vi "BuildPlaylist.vi"(3 "playlist":string="Current.txt") -> ()   [LabVIEW 2010]
uses:
  SlideParams.ctl
  <vilib>/Utility/file.llb/Read From Spreadsheet File (string).vi
  <vilib>/Utility/file.llb/Write To Spreadsheet File (string).vi
  <vilib>/Utility/cursorutil.llb/Set Cursor (Icon Pict).vi
panel:
  out "last last lineup":string[][](array[string])
  out "last lineup":string[][](array[string])
  out "Moving":bool
  in  "Revert":bool
  in  "Preview":bool
  in  "Save As":bool
  in  "Undo":bool
  out "location":cluster{dbl, dbl}
  out "Offset":cluster{"X":i32, "Y":i32}
  out "slide":i32
  in  "Tab Control":enum32{"Table", "Map", "LUT"}(tab)=enum."Map"
  in  "Table Control":string[][](table)
  out "Total":i32
  in  "ZOOM":dbl(slide) scale=0.1..2.0
  out "Slide":picture
  out "2D Map":picture
  in  "iterator":i32
  in  "Mod":T1=enum."Bounce"
  out "LUT":T2(array[cluster])
  in  "Save":bool
  # "/"
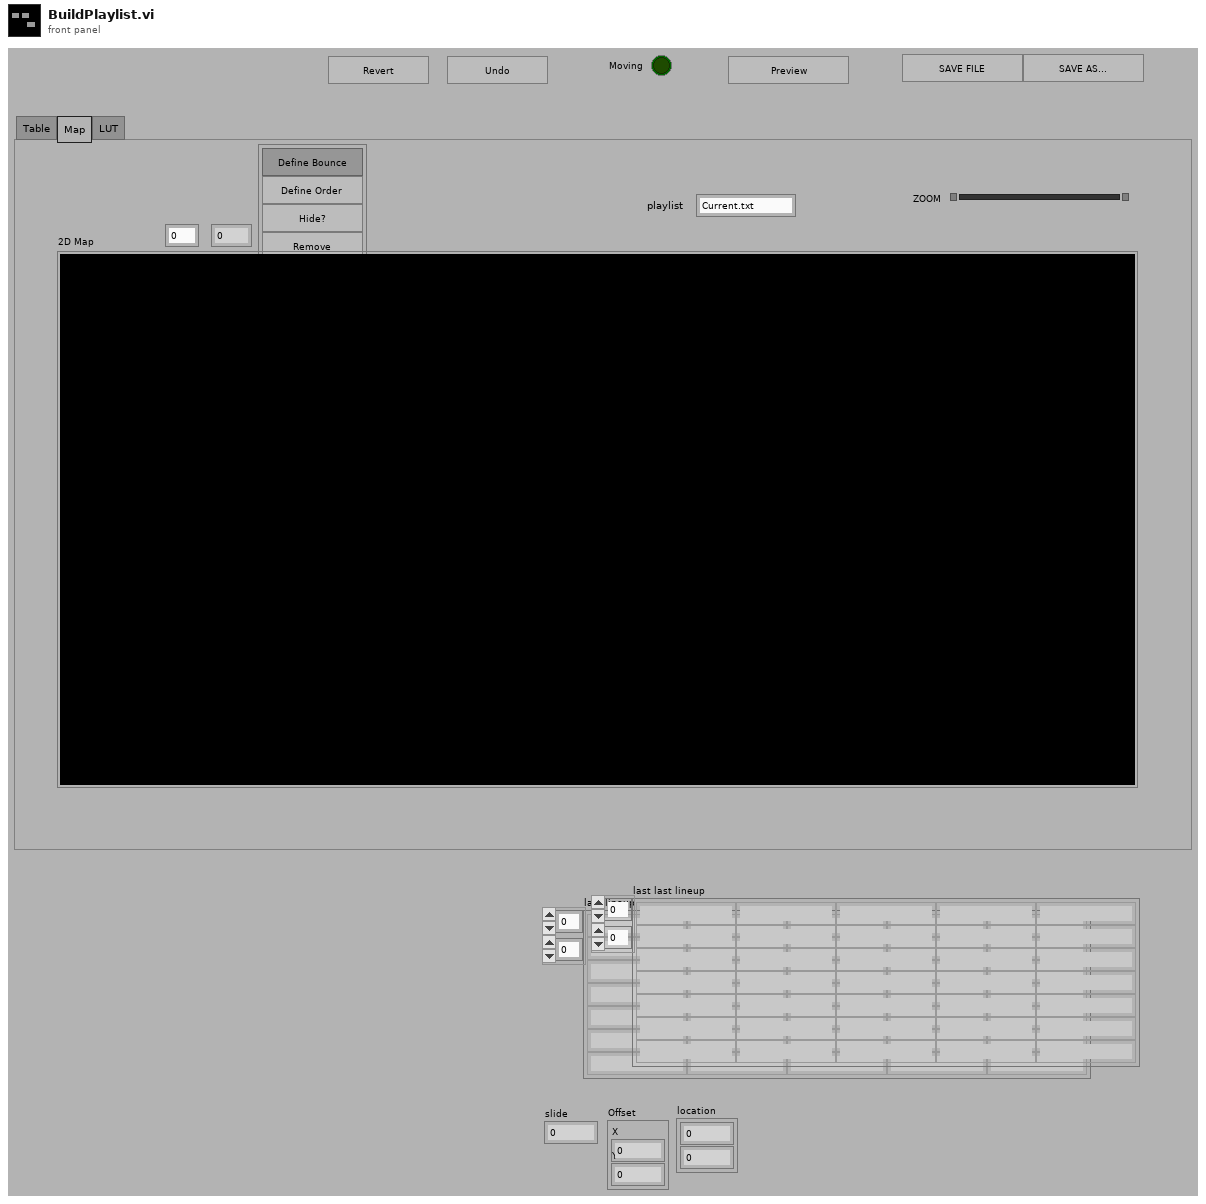
[diagram p1: front panel]
types:
  T1 = typedef "SlideParams.ctl" = enum32{"No Selection", "Bounce", "Order", "Hide", "Remove"}
  T2 = cluster{"col":i32, "row":i32, "rect":cluster{"left":i16, "top":i16, "right":i16, "bottom":i16}, "Name":string}[]
  T3 = typedef "LVPoint32TypeDef.ctl" = cluster{"Horizontal":i32, "Vertical":i32}
  T4 = typedef "LVMouseTypeDef.ctl" = cluster{"Mouse Position":cluster{"X":i32, "Y":i32}, "Mouse Modifiers":cluster{"Button Down":bool, "Shift Mod":bool, "Menu Mod":bool, "Option Mod":bool}}
  T5 = typedef "LVPointTypeDef.ctl" = cluster{"Horizontal":i16, "Vertical":i16}
  T6 = typedef "LVPositionTypeDef.ctl" = cluster{"Left":i32, "Top":i32}
  T7 = cluster{"col":i32, "row":i32, "rect":cluster{"left":i16, "top":i16, "right":i16, "bottom":i16}, "Name":string}
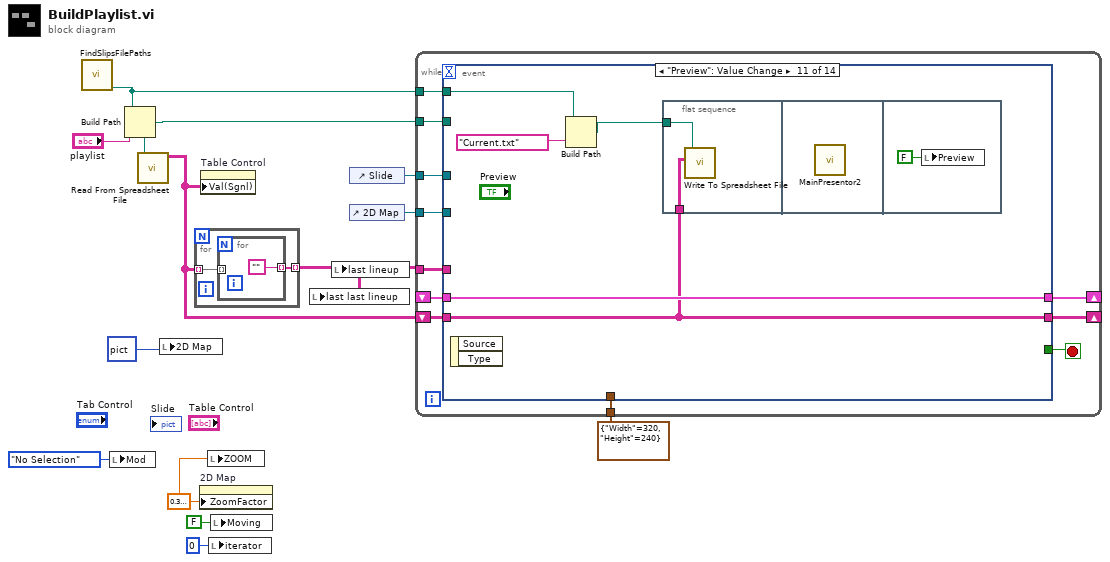
[diagram p0: block diagram]
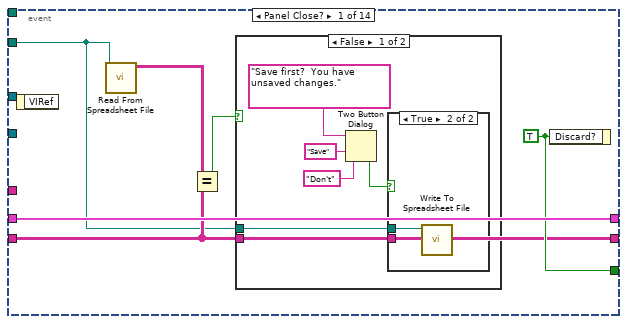
[diagram p2: hidden frame]
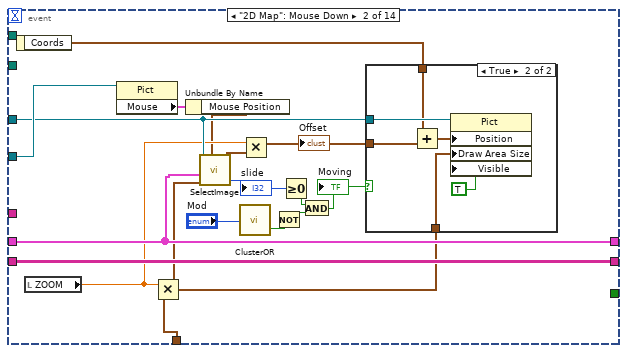
[diagram p5: hidden frame]
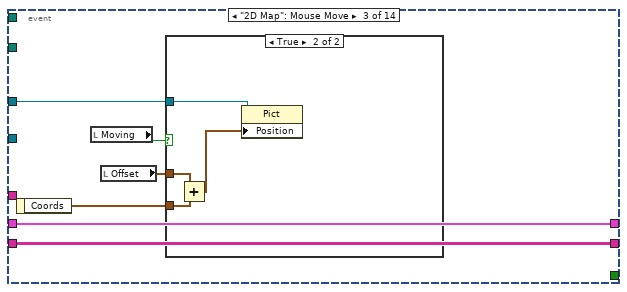
[diagram p7: hidden frame]
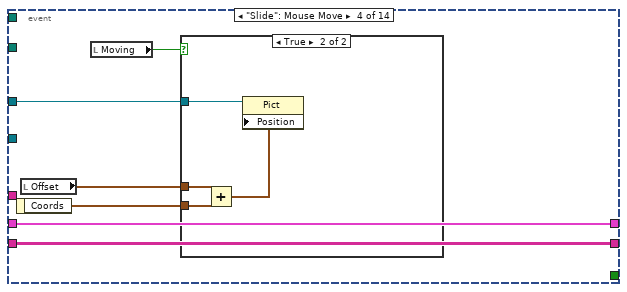
[diagram p9: hidden frame]
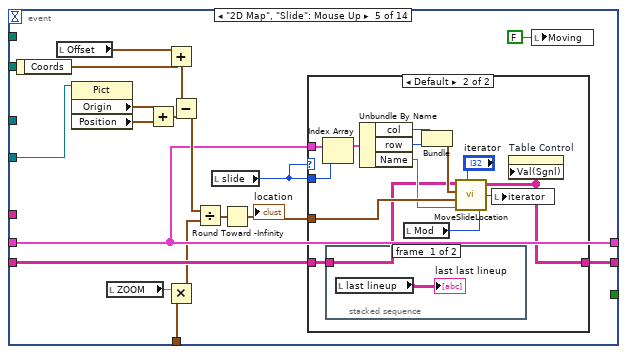
[diagram p11: hidden frame]
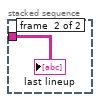
[diagram p13: hidden frame]
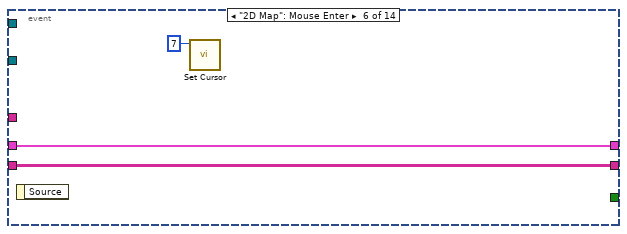
[diagram p14: hidden frame]
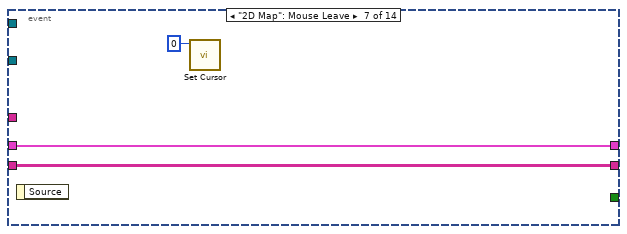
[diagram p15: hidden frame]
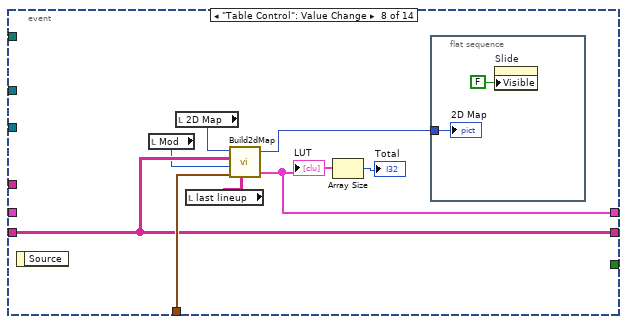
[diagram p16: hidden frame]
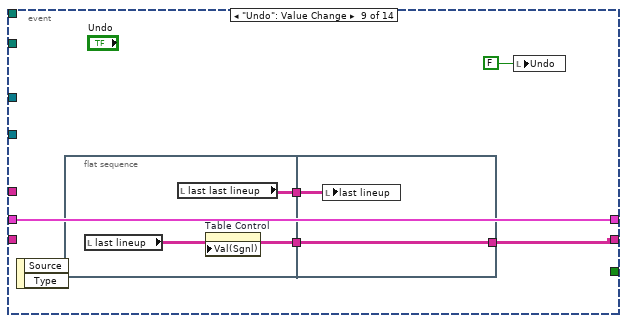
[diagram p17: hidden frame]
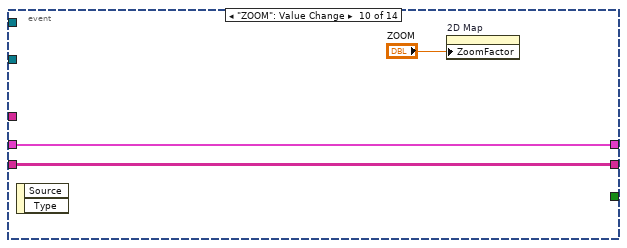
[diagram p18: hidden frame]
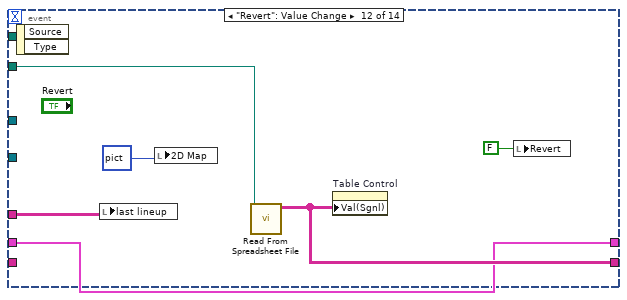
[diagram p19: hidden frame]
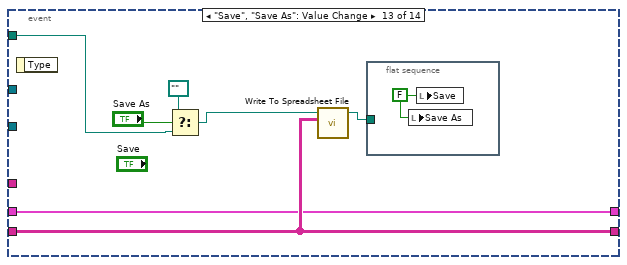
[diagram p20: hidden frame]
diagram:
  w8 = sgl 0.3 ("Zoom Factor")
  n1 = call "FindSlipsFilePaths.vi"() -> ("Playlists"=w1:path)  [unwired: 2 in, 4 out]
  n2 = local write "Mod"(SlideParams."No Selection" ("Mod")) -> ()
  n3 = Build Path(base path=w1, name or relative path="playlist") -> (appended path=w5:path)
  n4 = call-poly <vilib>:"Read From Spreadsheet File.vi"("file path (dialog if empty)"=w5) -> ("all rows"=w4:string[][])  [unwired: 6 in, 4 out]
  n5 = local write "2D Map"(picture data[5B] ("new picture")) -> ()
  n6 = for {
    tunnel: w4 -> [w15] mode=indexing
    tunnel: [w14] -> w2 mode=indexing
    n7 = for {
      tunnel: w15 -> [_] mode=indexing
      tunnel: [""] -> w14 mode=indexing
    }
  }
  n8 = property on="2D Map" class="Pict"("ZoomFactor"=w8) -> ()  [unwired: 2 in, 2 out]
  n9 = property on="Table Control" class="Tbl (strict)"("Val(Sgnl)"=w4) -> ()  [unwired: 2 in, 2 out]
  n10 = local write "ZOOM"(w8) -> ()
  n11 = local write "iterator"(0 ("iterator")) -> ()
  n12 = local write "Moving"(FALSE ("Moving")) -> ()
  n13 = local write "last last lineup"(w2) -> ()
  n14 = local write "last lineup"(w2) -> ()
  n15 = control-ref of="Slide"() -> (w10:refnum<vi>)
  n16 = control-ref of="2D Map"() -> (w11:refnum<vi>)
  n17 = while {
    tunnel: cluster{"Width":i32, "Height":i32} {"Width"=320, "Height"=240} ("Desired Dimensions") -> [w26]
    tunnel: w11 -> [w25]
    tunnel: w10 -> [w24]
    shift-right: [w22] -> _
    shift-left: w4 -> [w23]
    shift-right: [w21] -> _
    shift-left: _ -> [w20]
    tunnel: w1 -> [w19]
    tunnel: w5 -> [w18]
    tunnel: w2 -> [w17]
    stop <- w27 stop-if-true
    n18 = event shown="[10] \"Preview\": Value Change" {
      selector: _ -> [_ _ _ _ _ _ _ _ _ _ _ _ _ _]
      dyn-events: _ -> [_ _ _ _ _ _ _ _ _ _ _ _ _ _]
      timeout: _ -> [_ _ _ _ _ _ _ _ _ _ _ _ _ _]
      tunnel: [w30 _ _ _ _ _ _ _ _ _ _ _ _ _] -> w27
      tunnel: w26 -> [_ w56 _ _ w90 _ _ w133 _ _ _ _ _ _]
      tunnel: w25 -> [_ w59 _ _ w91 _ _ _ _ _ _ _ _ _]
      tunnel: w24 -> [_ w55 w68 w78 _ _ _ _ _ _ _ _ _ _]
      tunnel: w23 -> [w29 w58 w67 w77 w93 w121 w124 w132 _ w147 w148 _ w168 w171]
      tunnel: [w29 w58 w67 w77 w94 w121 w124 w132 w139 w147 w148 w160 w168 w170] -> w22
      tunnel: [w33 w57 w66 w76 w92 w120 w123 w129 w140 w146 w152 w159 w167 w173] -> w21
      tunnel: w20 -> [w33 w57 w66 w76 w92 w120 w123 _ w140 w146 w152 w159 w167 w173]
      tunnel: w19 -> [_ _ _ _ _ _ _ _ _ _ w151 _ _ _]
      tunnel: w18 -> [w28 _ _ _ _ _ _ _ _ _ _ w161 w163 _]
      tunnel: w17 -> [_ _ _ _ _ _ _ _ _ _ _ w157 _ _]
      event Panel Close? {
        w30 = TRUE ("Discard?")
        n19 = event-data() -> ()  [unwired: 1 in, 1 out]
        n20 = call-poly <vilib>:"Read From Spreadsheet File.vi"("file path (dialog if empty)"=w28) -> ("all rows"=w32:string[][])  [unwired: 6 in, 4 out]
        n21 = Equal?(x=w32, y=w29) -> (x = y?=w31:bool)
        n22 = case shown="False" w31 {
          tunnel: w29 -> [w35 _]
          tunnel: w28 -> [w34 _]
          frame False {
            n23 = Two Button Dialog(message="Save first?  You have unsaved changes.", 1:"Don't" ("T button name (\"OK\")"), 2:"Save" ("T button name (\"OK\")")) -> (T button?=w36:bool)
            n24 = case shown="True" w36 {
              tunnel: w35 -> [_ w41]
              tunnel: w34 -> [_ w40]
              frame False {
              }
              frame True {
                n25 = call-poly <vilib>:"Write To Spreadsheet File.vi"("2D data"=w41, "file path (dialog if empty)"=w40) -> ()  [unwired: 6 in, 1 out]
              }
            }
          }
          frame True {
          }
        }
        n26 = event-data("Discard?"=w30) -> ()  [unwired: 1 in, 1 out]
      }
      event "2D Map": Mouse Down {
        n27 = event-data() -> ("Coords"=w54:T3)  [unwired: 1 in]
        n28 = local read "ZOOM"() -> (w53:dbl)
        n29 = property on="Property Node" class="Pict"(reference=w59) -> ("Mouse"=w52:T4)  [unwired: 1 in, 2 out]
        n30 = Multiply(x=w53, y=w56) -> (x*y=w49:cluster{"Width":dbl, "Height":dbl})
        n31 = Unbundle By Name(w52) -> ("Mouse Position"=w50:cluster{"X":i32, "Y":i32})
        n32 = call "SelectImage.vi"("Selected Slide"=w55, "LUT"=w57, "Desired Dimensions"=w49, "Mouse Position"=w50) -> ("Offset"=w48:cluster{"X":i32, "Y":i32}, "slide"=w51:i32)  [unwired: 1 in, 1 out]
        "slide" <- w51
        n33 = call "ClusterOR.vi"("Mod"="Mod") -> ("selection?"=w42:bool)  [unwired: 1 out]
        n34 = Multiply(x=w53, y=w48) -> (x*y=w47:cluster{"X":dbl, "Y":dbl})
        "Offset" <- w47
        n35 = Not(x=w42) -> (.not. x?=w46:bool)
        n36 = Greater Or Equal To 0?(x=w51) -> (x >= 0?=w45:bool)
        n37 = And(x=w45, y=w46) -> (x .and. y?=w44:bool)
        "Moving" <- w44
        n38 = case shown="True" w44 {
          tunnel: w55 -> [_ w65]
          tunnel: w49 -> [_ w64]
          tunnel: w47 -> [_ w63]
          tunnel: w54 -> [_ w62]
          frame False {
          }
          frame True {
            n39 = Add(x=w62, y=w63) -> (x+y=w61:cluster{dbl, dbl})
            n40 = property class="Pict"(reference=w65, "Position"=w61, "Draw Area Size"=w64, "Visible"=TRUE) -> ()  [unwired: 1 in, 2 out]
          }
        }
      }
      event "2D Map": Mouse Move {
        n41 = event-data() -> ("Coords"=w70:T3)  [unwired: 1 in]
        n42 = local read "Moving"() -> (w71:bool)
        n43 = local read "Offset"() -> (w69:cluster{"X":i32, "Y":i32})
        n44 = case shown="True" w71 {
          tunnel: w70 -> [_ w75]
          tunnel: w69 -> [_ w74]
          tunnel: w68 -> [_ w73]
          frame False {
          }
          frame True {
            n45 = Add(x=w74, y=w75) -> (x+y=w72:T3)
            n46 = property class="Pict"(reference=w73, "Position"=w72) -> ()  [unwired: 1 in, 2 out]
          }
        }
      }
      event "Slide": Mouse Move {
        n47 = event-data() -> ("Coords"=w80:T3)  [unwired: 1 in]
        n48 = local read "Offset"() -> (w79:cluster{"X":i32, "Y":i32})
        n49 = local read "Moving"() -> (w81:bool)
        n50 = case shown="True" w81 {
          tunnel: w80 -> [_ w85]
          tunnel: w79 -> [_ w84]
          tunnel: w78 -> [_ w83]
          frame False {
          }
          frame True {
            n51 = Add(x=w84, y=w85) -> (x+y=w82:T3)
            n52 = property class="Pict"(reference=w83, "Position"=w82) -> ()  [unwired: 1 in, 2 out]
          }
        }
      }
      event "2D Map", "Slide": Mouse Up {
        n53 = event-data() -> ("Coords"=w102:T3)  [unwired: 1 in]
        n54 = local read "Offset"() -> (w87:cluster{"X":i32, "Y":i32})
        n55 = property class="Pict"(reference=w91) -> ("Origin"=w100:T5, "Position"=w99:T6)  [unwired: 1 in, 2 out]
        n56 = local read "ZOOM"() -> (w88:dbl)
        n57 = Add(x=w100, y=w99) -> (x+y=w98:T6)
        n58 = Add(x=w87, y=w102) -> (x+y=w97:T3)
        n59 = Multiply(x=w88, y=w90) -> (x*y=w89:cluster{"Width":dbl, "Height":dbl})
        n60 = Subtract(x=w97, y=w98) -> (x-y=w96:T3)
        n61 = Divide(x=w96, y=w89) -> (x/y=w101:cluster{dbl, dbl})
        n62 = local read "slide"() -> (w86:i32)
        n63 = Round Toward -Infinity(1:w101) -> (0:w95:cluster{dbl, dbl})
        "location" <- w95
        n64 = case shown="Default" w86 {
          tunnel: w95 -> [_ w117]
          tunnel: w86 -> [_ w116]
          tunnel: [w104 w110] -> w94
          tunnel: w93 -> [w104 w105]
          tunnel: w92 -> [_ w109]
          frame -1 {
          }
          frame Default {
            n65 = Index Array(array=w109, index=w116) -> (element=w115:T7)
            n66 = stacked-sequence {
              tunnel: w105 -> [_ w119]
              frame #0 {
                n67 = local read "last lineup"() -> (→"last last lineup":string[][])
              }
              frame #1 {
                "last lineup" <- w119
              }
            }
            n68 = Unbundle By Name(w115) -> ("col"=w113:i32, "row"=w112:i32, "Name"=w114:string)
            n69 = local read "Mod"() -> (w108:T1)
            n70 = Bundle("col"=w113, "row"=w112) -> (w111:cluster{"col":i32, "row":i32})  [unwired: 1 in]
            n71 = call "MoveSlideLocation.vi"("old Table"=w105, "start location"=w111, "end location"=w117, "name"=w114, "order #"="iterator", "Mod"=w108) -> ("new Table"=w110:string[][], "iterator"=w106:i32)
            n72 = local write "iterator"(w106) -> ()
            n73 = property on="Table Control" class="Tbl (strict)"("Val(Sgnl)"=w110) -> ()  [unwired: 2 in, 2 out]
          }
        }
        n74 = local write "Moving"(FALSE ("Moving")) -> ()
      }
      event "2D Map": Mouse Enter {
        n75 = event-data() -> ()  [unwired: 1 in, 1 out]
        n76 = call-poly <vilib>:"Set Cursor.vi"("icon"=u16 7) -> ()  [unwired: 9 in, 2 out]
      }
      event "2D Map": Mouse Leave {
        n77 = event-data() -> ()  [unwired: 1 in, 1 out]
        n78 = call-poly <vilib>:"Set Cursor.vi"("icon"=u16 0) -> ()  [unwired: 9 in, 2 out]
      }
      event "Table Control": Value Change {
        n79 = event-data() -> ()  [unwired: 1 in, 1 out]
        n80 = local read "Mod"() -> (w128:T1)
        n81 = local read "2D Map"() -> (w127:picture)
        n82 = local read "last lineup"() -> (w126:string[][])
        n83 = call "Build2dMap.vi"("2D in"=w127, "new listing"=w132, "Mod"=w128, "Desired Dimensions"=w133, "Old listing"=w126) -> ("2D Map"=w131:picture, "LUT"=w129:T2)  [unwired: 1 out]
        "LUT" <- w129
        n84 = Array Size(array=w129) -> (size(s)=→"Total":i32)
        n85 = flat-sequence {
          tunnel: w131 -> [w135]
          frame #0 {
            n86 = property on="Slide" class="Pict"("Visible"=FALSE) -> ()  [unwired: 2 in, 2 out]
            "2D Map" <- w135
          }
        }
      }
      event "Undo": Value Change {
        n87 = event-data() -> ()  [unwired: 1 in, 2 out]
        n88 = flat-sequence {
          tunnel: [w142] -> w137
          tunnel: [w141] -> w136
          tunnel: [w144] -> w139
          tunnel: w137 -> [w144]
          tunnel: w136 -> [w143]
          frame #0 {
            n89 = local read "last lineup"() -> (w142:string[][])
            n90 = local read "last last lineup"() -> (w141:string[][])
            n91 = property on="Table Control" class="Tbl (strict)"("Val(Sgnl)"=w142) -> ()  [unwired: 2 in, 2 out]
          }
          frame #1 {
            n92 = local write "last lineup"(w143) -> ()
          }
        }
        n93 = local write "Undo"(FALSE ("Undo")) -> ()
      }
      event "ZOOM": Value Change {
        n94 = event-data() -> ()  [unwired: 1 in, 2 out]
        n95 = property on="2D Map" class="Pict"("ZoomFactor"="ZOOM") -> ()  [unwired: 2 in, 2 out]
      }
      event "Preview": Value Change {
        n96 = event-data() -> ()  [unwired: 1 in, 2 out]
        n97 = Build Path(base path=w151, name or relative path="Current.txt") -> (appended path=w149:path)
        n98 = flat-sequence {
          tunnel: w149 -> [w154]
          tunnel: w148 -> [w153]
          frame #0 {
            n99 = call-poly <vilib>:"Write To Spreadsheet File.vi"("2D data"=w153, "file path (dialog if empty)"=w154) -> ()  [unwired: 6 in, 1 out]
          }
          frame #1 {
            n100 = call "MainPresentor2.vi"() -> ()  [unwired: 12 in]
          }
          frame #2 {
            n101 = local write "Preview"(FALSE ("Preview")) -> ()
          }
        }
      }
      event "Revert": Value Change {
        n102 = event-data() -> ()  [unwired: 1 in, 2 out]
        n103 = local write "last lineup"(w157) -> ()
        n104 = local write "2D Map"(picture data[5B] ("new picture")) -> ()
        n105 = call-poly <vilib>:"Read From Spreadsheet File.vi"("file path (dialog if empty)"=w161) -> ("all rows"=w160:string[][])  [unwired: 6 in, 4 out]
        n106 = property on="Table Control" class="Tbl (strict)"("Val(Sgnl)"=w160) -> ()  [unwired: 2 in, 2 out]
        n107 = local write "Revert"(FALSE ("Revert")) -> ()
      }
      event "Save", "Save As": Value Change {
        n108 = event-data() -> ()  [unwired: 1 in, 1 out]
        n109 = Select(t=path "", s="Save As", f=w163) -> (s? t:f=w165:path)
        n110 = call-poly <vilib>:"Write To Spreadsheet File.vi"("2D data"=w168, "file path (dialog if empty)"=w165) -> ("new file path (Not A Path if cancelled)"=w162:path)  [unwired: 6 in]
        n111 = flat-sequence {
          tunnel: w162 -> [_]
          frame #0 {
            w169 = FALSE ("Save")
            n112 = local write "Save As"(w169) -> ()
            n113 = local write "Save"(w169) -> ()
          }
        }
      }
      event Menu Selection (User) {
        n114 = event-data() -> ("ItemTag"=w172:string)  [unwired: 1 in]
        n115 = case shown="\"AddSlide\"" w172 {
          tunnel: w171 -> [w174 w175 w177 w179 w181 w183 w186 w194]
          tunnel: [w174 w175 w177 w179 w181 w183 w185 w193] -> w170
          frame Default {
          }
          frame "Preview" {
            n116 = property on="Preview" class="Bool (strict)"("Val(Sgnl)"=TRUE) -> ()  [unwired: 2 in, 2 out]
          }
          frame "Save" {
            n117 = property on="Save" class="Bool (strict)"("Val(Sgnl)"=TRUE) -> ()  [unwired: 2 in, 2 out]
          }
          frame "SaveAs" {
            n118 = property on="Save As" class="Bool (strict)"("Val(Sgnl)"=TRUE) -> ()  [unwired: 2 in, 2 out]
          }
          frame "Revert" {
            n119 = property on="Revert" class="Bool (strict)"("Val(Sgnl)"=TRUE) -> ()  [unwired: 2 in, 2 out]
          }
          frame "Undo" {
            n120 = property on="Undo" class="Bool (strict)"("Val(Sgnl)"=TRUE) -> ()  [unwired: 2 in, 2 out]
          }
          frame "NewSlide" {
            n121 = call "SelectTemplate.vi"() -> ("Success"=w188:bool, "name"=w187:string)  [unwired: 2 in]
            n122 = case shown="True" w188 {
              tunnel: w187 -> [_ w190]
              tunnel: w186 -> [w189 w192]
              tunnel: [w189 w191] -> w185
              frame False {
              }
              frame True {
                n123 = call "OpenSlide.vi"("Slide"=w190) -> ()
                n124 = local write "last lineup"(w192) -> ()
                n125 = call "AddNewSlideIntoListing.vi"("Old Listing"=w192, "name"=w190) -> ("New listing"=w191:string[][])
                n126 = property on="Table Control" class="Tbl (strict)"("Val(Sgnl)"=w191) -> ()  [unwired: 2 in, 2 out]
              }
            }
          }
          frame "AddSlide" {
            n127 = call "SelectSlide.vi"() -> ("Success"=w196:bool, "name"=w195:string)  [unwired: 2 in]
            n128 = case shown="True" w196 {
              tunnel: w195 -> [_ w198]
              tunnel: w194 -> [w197 w200]
              tunnel: [w197 w199] -> w193
              frame False {
              }
              frame True {
                n129 = call "OpenSlide.vi"("Slide"=w198) -> ()
                n130 = local write "last lineup"(w200) -> ()
                n131 = call "AddNewSlideIntoListing.vi"("Old Listing"=w200, "name"=w198) -> ("New listing"=w199:string[][])
                n132 = property on="Table Control" class="Tbl (strict)"("Val(Sgnl)"=w199) -> ()  [unwired: 2 in, 2 out]
              }
            }
          }
        }
      }
    }
  }
